vi "RT Loop - System Health and FPGA Monitoring.vi"(11 "Message Queue":refnum<queue> caption="消息队列") -> ()   [LabVIEW 2013]
uses:
  support/Message Queue/Message Cluster.ctl
  controls/FPGA VI Reference.ctl
  <vilib>/nisyscfg/Close (System).vi
  Globals/Global - All RT Loop Stop.vi
  Globals/Global - Monitoring Variables.vi
  Globals/Global - Configuration Options.vi
  <vilib>/Utility/error.llb/Error Cluster From Error Code.vi
  <vilib>/rvi/errors/niLvFpgaAdjustHostInterfaceError.vi
  <vilib>/rvi/interface/nirviReadWriteControl/nirviReadWriteControl.xnode
  FPGA Bitfiles/LabVIEWFPGAWavef_FPGA_FPGAMain_vTbN89OLNVY.lvbitx
  FPGA Main.vi
  <vilib>/nisyscfg/nisyscfg.lvlib
  <resource>/objmgr/nisysapi.rc
  <vilib>/NI_Real-Time Target Support.lvlib
  NiFpgaLv.dll
  support/Message Queue/Message Queue.lvlib
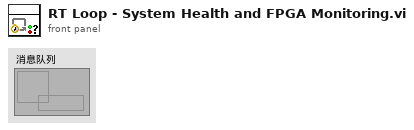
[diagram p1: front panel]
types:
  T1 = typedef "FPGA VI Reference.ctl" = refnum<k20>
  T2 = typedef "NI_Real-Time Target Support.lvlib/RT CPU Load.ctl" = cluster{"Total (%)":dbl, "Time Critical (%)":dbl, "Timed Structures (%)":dbl, "High (%)":dbl, "Above Normal (%)":dbl, "Normal (%)":dbl, "Background (%)":dbl, "Idle (%)":dbl, "ISR (%)":dbl}
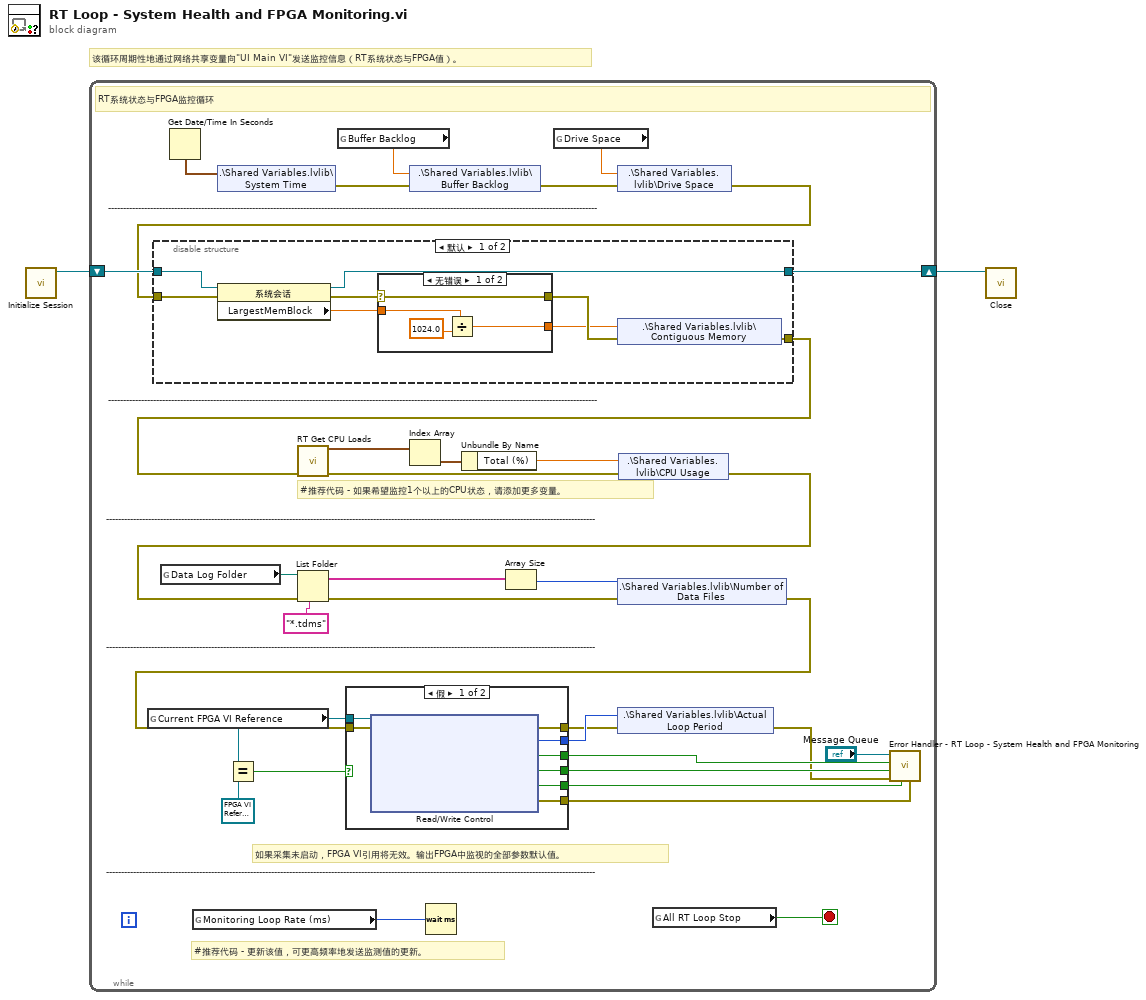
[diagram p0: block diagram]
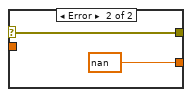
[diagram p2: hidden frame]
diagram:
  # "该循环周期性地通过网络共享变量向\"UI Main VI\"发送监控信息（RT系统状态与FPGA值）。"
  n1 = call <vilib>:"Initialize Session.vi"() -> ("session out"=w2:refnum<k21>)  [unwired: 10 in, 1 out]
  n2 = while {
    shift-right: [w19] -> w1
    shift-left: w2 -> [w20]
    stop <- w32 stop-if-true
    # "-------------------------------------------------------------------------------------------------------------------------------------------------------------------"
    # "-------------------------------------------------------------------------------------------------------------------------------------------------------------------"
    # "-------------------------------------------------------------------------------------------------------------------------------------------------------------------"
    # "-------------------------------------------------------------------------------------------------------------------------------------------------------------------"
    # "-------------------------------------------------------------------------------------------------------------------------------------------------------------------"
    # "#推荐代码 - 如果希望监控1个以上的CPU状态，请添加更多变量。"
    # "#推荐代码 - 更新该值，可更高频率地发送监测值的更新。"
    # "如果采集未启动，FPGA VI引用将无效。输出FPGA中监视的全部参数默认值。"
    # "RT系统状态与FPGA监控循环"
    n3 = global read "Global - Monitoring Variables.vi" "Current FPGA VI Reference"() -> (w18:T1)
    n4 = global read "Global - Configuration Options.vi" "Data Log Folder"() -> (w6:path)
    n5 = Get Date/Time In Seconds() -> (seconds since 1Jan1904=w11:timestamp)
    n6 = global read "Global - Configuration Options.vi" "Monitoring Loop Rate (ms)"() -> (w7:u32)
    n7 = shared-variable ".\\Shared Variables.lvlib\\System Time"(w11) -> (error out=w5:errorcluster)  [unwired: 1 in]
    n8 = Equal?(x=w18, y=T1 refnum ("Current FPGA VI Reference")) -> (x = y?=w25:bool)
    n9 = global read "Global - Monitoring Variables.vi" "Buffer Backlog"() -> (w10:dbl)
    n10 = shared-variable ".\\Shared Variables.lvlib\\Buffer Backlog"(w10, error in=w5) -> (error out=w13:errorcluster)
    n11 = Wait (ms)(milliseconds to wait=w7) -> ()  [unwired: 1 out]
    n12 = global read "Global - Monitoring Variables.vi" "Drive Space"() -> (w12:dbl)
    n13 = shared-variable ".\\Shared Variables.lvlib\\Drive Space"(w12, error in=w13) -> (error out=w4:errorcluster)
    n14 = disable-structure shown="默认" {
      disable-tunnel: w20 -> [w41 w50]
      disable-tunnel: [w40 w50] -> w19
      disable-tunnel: w4 -> [w37 w51]
      disable-tunnel: [w36 w51] -> w3
      frame condition #0 (active) {
        n15 = property class="系统会话"(reference=w41, error in=w37) -> (reference out=w40:refnum<k21>, error out=w42:errorcluster, "LargestMemBlock"=w38:dbl)
        n16 = case shown="无错误" w42 {
          selector: w42 -> [w46 w48]
          tunnel: w38 -> [w45 _]
          tunnel: [w47 nan] -> w39
          tunnel: [w46 w48] -> w43
          frame No Error {
            # "将千字节转换为字节"
            n17 = Divide(x=w45, y=1024.0 ("x")) -> (x/y=w47:dbl)
          }
          frame Error {
            # "不支持的属性。"
          }
        }
        n18 = shared-variable ".\\Shared Variables.lvlib\\Contiguous Memory"(w39, error in=w43) -> (error out=w36:errorcluster)
      }
      frame condition #1 {
      }
    }
    n19 = call <vilib>:"RT Get CPU Loads.vi"("error in (no error)"=w3) -> ("error out"=w35:errorcluster, "CPU loads"=w34:T2[])  [unwired: 9 in]
    n20 = Index Array(array=w34) -> (element=w33:T2)  [unwired: 1 in]
    n21 = Unbundle By Name(w33) -> ("Total (%)"=w24:dbl)
    n22 = shared-variable ".\\Shared Variables.lvlib\\CPU Usage"(w24, error in=w35) -> (error out=w17:errorcluster)
    n23 = List Folder(path=w6, pattern="*.tdms", error in=w17) -> (filenames=w22:string[], error out=w16:errorcluster)  [unwired: 1 in, 2 out]
    n24 = Array Size(array=w22) -> (size(s)=w21:i32)
    n25 = shared-variable ".\\Shared Variables.lvlib\\Number of Data Files"(w21, error in=w16) -> (error out=w15:errorcluster)
    n26 = case shown="假" w25 {
      tunnel: [w59 _] -> w14
      tunnel: [w58 _] -> w31
      tunnel: [w57 _] -> w30
      tunnel: [w56 _] -> w29
      tunnel: [w55 _] -> w28
      tunnel: [w54 _] -> w27
      tunnel: w18 -> [w53 _]
      tunnel: w15 -> [w52 _]
      frame False {
        n27 = xnode "Read/Write Control"("FPGA VI引用输入"=w53, "错误输入"=w52) -> ("错误输出"=w59:errorcluster, "Actual Loop Period (ticks)"=w58:u32, "Module Underflow"=w57:bool, "DMA FIFO Full"=w56:bool, "Different Channel Count"=w55:bool, "FPGA Error"=w54:errorcluster)  [unwired: 1 out]
      }
      frame True {
      }
    }
    n28 = shared-variable ".\\Shared Variables.lvlib\\Actual Loop Period"(w31, error in=w14) -> (error out=w8:errorcluster)
    n29 = global read "Global - All RT Loop Stop.vi" "All RT Loop Stop"() -> (w32:bool)
    n30 = call "Error Handler - RT Loop - System Health and FPGA Monitoring.vi"("FPGA Error (FPGA)"=w27, "Different Channel Count (FPGA)"=w28, "error in (no error)"=w8, "DMA FIFO Full (FPGA)"=w29, "Module Underflow (FPGA)"=w30, "Message Queue"="Message Queue") -> ()  [unwired: 5 in, 1 out]
  }
  n31 = call-poly <vilib>:"Close.vi"("session in"=w1) -> ()  [unwired: 10 in, 1 out]
